vi "Phasor Check Calibration Map Change.vi"(9 "Phasor Calibration Map 2":T1={"Phasor Frequency"=80000000.0, "Calibration Lifetime"=1e-09, "ROI Centers"=[], "ROI Descriptors"=[], "Map Resolution X"=0, "Map Resolution Y"=0, "z Array"=[]} {"ROI Descriptors"."Contours"."Type" items=["No Selection", "Point", "Line", "Rectangle", "Oval", "Polygon", "Freehand Region", "Annulus", "Unused2", "Unused3", "Broken Line", "Freehand Line", "Rotated Rectangle"]}, 11 "Phasor Calibration Map 1":T1={"Phasor Frequency"=80000000.0, "Calibration Lifetime"=1e-09, "ROI Centers"=[], "ROI Descriptors"=[], "Map Resolution X"=0, "Map Resolution Y"=0, "z Array"=[]} {"ROI Descriptors"."Contours"."Type" items=["No Selection", "Point", "Line", "Rectangle", "Oval", "Polygon", "Freehand Region", "Annulus", "Unused2", "Unused3", "Broken Line", "Freehand Line", "Rotated Rectangle"]}) -> (3 "Changed?":bool, 6 "elapsed (relative) seconds":dbl)   [LabVIEW 2021, in "Phasor.lvlib"]
uses:
  Phasor.lvlib
  Phasor Calibration Map v2.ctl
  <userlib>/_OpenG.lib/array/array.llb/Filter 1D Array with Scalar (CDB)__ogtk.vi
  Time/Time.lvlib
  <userlib>/_OpenG.lib/array/array.llb/openg_array.lvlib
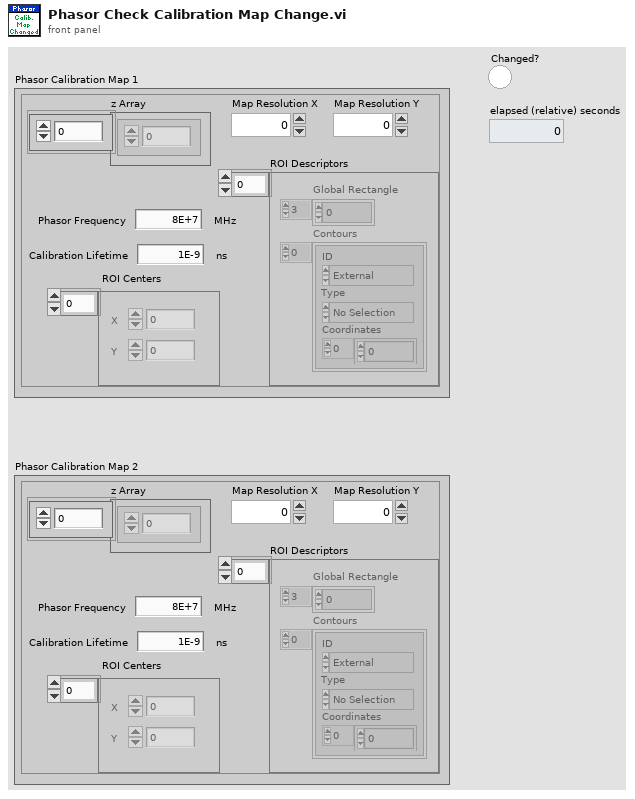
[diagram p1: front panel]
types:
  T1 = typedef "Phasor.lvlib/Phasor Calibration Map v2.ctl" = cluster{"Phasor Frequency":dbl[unit], "Calibration Lifetime":dbl[unit], "ROI Centers":cluster{"X":i32, "Y":i32}[], "ROI Descriptors":T2[], "Map Resolution X":i32, "Map Resolution Y":i32, "z Array":cdb[]}
  T2 = typedef "ROI Descriptor" = cluster{"Global Rectangle":i32[], "Contours":cluster{"ID":enum32{"External", "Internal"}, "Type":u32, "Coordinates":i32[]}[]}
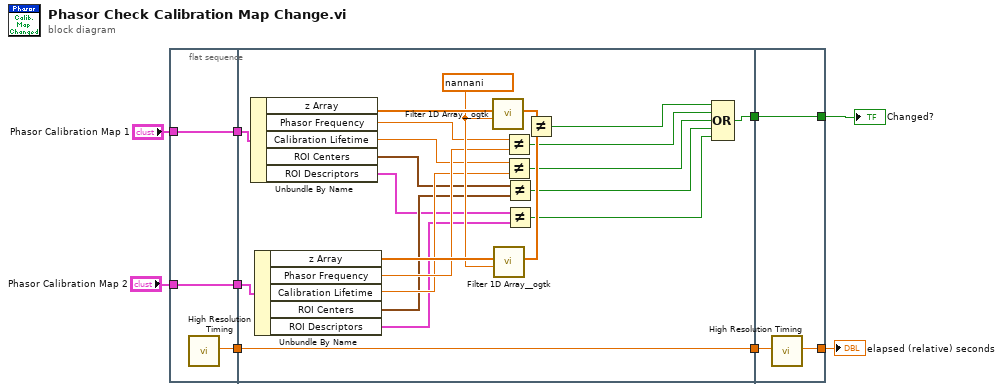
[diagram p0: block diagram]
diagram:
  n1 = flat-sequence {
    tunnel: "Phasor Calibration Map 2" -> [w11]
    tunnel: "Phasor Calibration Map 1" -> [w12]
    tunnel: [w12] -> w6
    tunnel: [w11] -> w5
    tunnel: [w10] -> w2
    tunnel: w6 -> [w34]
    tunnel: w5 -> [w33]
    tunnel: [w15] -> w4
    tunnel: [w13] -> w3
    tunnel: w2 -> [w13]
    tunnel: [w37] -> w7
    tunnel: w4 -> [w37]
    tunnel: w3 -> [w36]
    tunnel: [w35] -> w1
    frame #0 {
      n2 = call "High Resolution Timing.vi"() -> ("elapsed (relative) seconds"=w10:dbl)  [unwired: 17 in, 2 out]
    }
    frame #1 {
      w30 = cdb nan+nani ("Element(s) to Remove")
      n3 = Unbundle By Name(w34) -> ("z Array"=w31:cdb[], "Phasor Frequency"=w26:dbl[unit], "Calibration Lifetime"=w23:dbl[unit], "ROI Centers"=w20:cluster{"X":i32, "Y":i32}[], "ROI Descriptors"=w18:T2[])
      n4 = Unbundle By Name(w33) -> ("z Array"=w32:cdb[], "Phasor Frequency"=w25:dbl[unit], "Calibration Lifetime"=w22:dbl[unit], "ROI Centers"=w19:cluster{"X":i32, "Y":i32}[], "ROI Descriptors"=w14:T2[])
      n5 = call-poly <userlib>:"Filter 1D Array__ogtk.vi"("items to filter"=w30, "array"=w31) -> ("filtered array"=w29:cdb[])  [unwired: 4 in, 1 out]
      n6 = call-poly <userlib>:"Filter 1D Array__ogtk.vi"("items to filter"=w30, "array"=w32) -> ("filtered array"=w28:cdb[])  [unwired: 4 in, 1 out]
      n7 = Not Equal?(x=w26, y=w25) -> (x != y?=w24:bool)
      n8 = Not Equal?(x=w23, y=w22) -> (x != y?=w21:bool)
      n9 = Not Equal?(x=w20, y=w19) -> (x != y?=w17:bool)
      n10 = Not Equal?(x=w18, y=w14) -> (x != y?=w16:bool)
      n11 = Not Equal?(x=w29, y=w28) -> (x != y?=w27:bool)
      n12 = Compound Arithmetic op=OR(w27, w24, w21, w17, w16) -> (w15:bool)
    }
    frame #2 {
      n13 = call "High Resolution Timing.vi"("relative seconds (NaN)"=w36) -> ("elapsed (relative) seconds"=w35:dbl)  [unwired: 16 in, 2 out]
    }
  }
  "Changed?" <- w7
  "elapsed (relative) seconds" <- w1
